vi "NI VeriStand - Not a Ref.vi"(8 "error in (no error)":errorcluster, 11 "Item Ref":T1=18446744073709551615 format="%.0x") -> (0 "error out":errorcluster, 2 "Not a Ref":bool, 3 "Item Ref out":T1=18446744073709551615 format="%.0x")   [LabVIEW 2020, in "Custom Device Utility Library.lvlib"]
doc: "Gets whether the <B>Item Ref</B> you specify is a valid reference."
uses:
  <vilib>/NI VeriStand/Custom Device Tools/Custom Device Utility Library/Custom Device Utility Library.lvlib
  <vilib>/NI VeriStand/Custom Device API/Custom Device Item Ref.ctl
  <vilib>/NI VeriStand/Custom Device Tools/Custom Device Utility Library/NI VeriStand - Ref Constants.vi
  <vilib>/NI VeriStand/Custom Device API/Custom Device API.lvlib
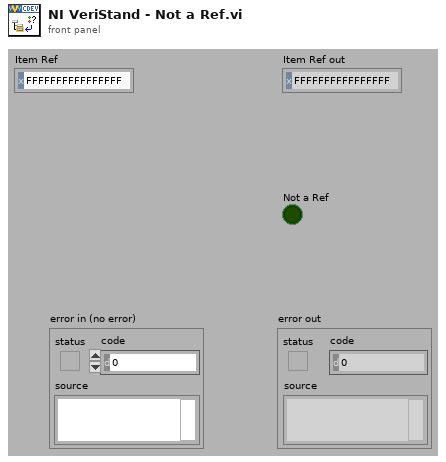
[diagram p1: front panel]
types:
  T1 = typedef "Custom Device API.lvlib/Custom Device Item Ref.ctl" = u64
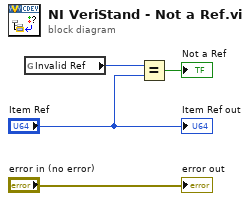
[diagram p0: block diagram]
diagram:
  n1 = global read "NI VeriStand - Ref Constants.vi" "Invalid Ref"() -> (w4:T1)
  n2 = Equal?(x=w4, y="Item Ref") -> (x = y?=→"Not a Ref":bool)
  "error out" <- "error in (no error)"
  "Item Ref out" <- "Item Ref"
